vi "Add Bad Input Error.vi"(4 "missing value":string, 6 "name":string, 8 "error in":errorcluster, 10 "in connections map":bool) -> (0 "error out":errorcluster)   [LabVIEW 2020, in "MeasurementLink Session Management.lvlib" / "Session Reservation.lvclass"]
uses:
  Session Reservation.lvclass
  MeasurementLink Measurement Server/Helpers/Error Strings Global Internal.vi
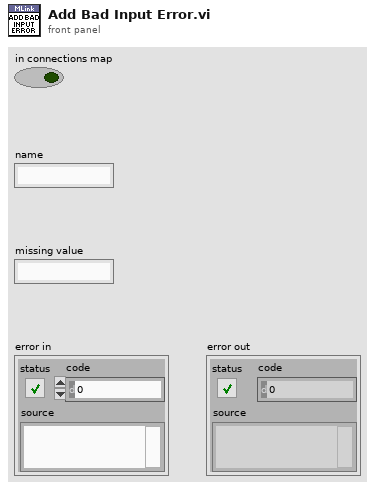
[diagram p1: front panel]
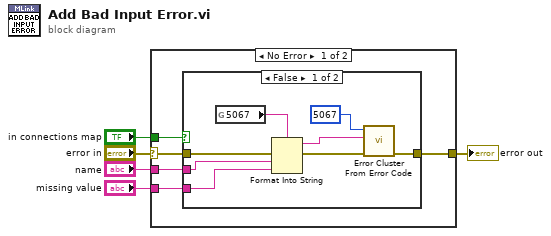
[diagram p0: block diagram]
diagram:
  n1 = case shown="No Error" "error in" {
    selector: "error in" -> [w8 w20]
    tunnel: "missing value" -> [w10 _]
    tunnel: "in connections map" -> [w9 _]
    tunnel: [w7 w20] -> w2
    tunnel: "name" -> [w6 _]
    frame No Error {
      n2 = case shown="False" w9 {
        tunnel: [w18 w19] -> w7
        tunnel: w8 -> [w16 w19]
        tunnel: w10 -> [w12 _]
        tunnel: w6 -> [w11 _]
        frame False {
          n3 = global read "Error Strings Global Internal.vi" "5067"() -> (w17:string)
          n4 = Format Into String(format string=w17, error in=w16, w11, w12) -> (resulting string=w13:string, error out=w15:errorcluster)  [unwired: 1 in]
          n5 = call <vilib>:"Error Cluster From Error Code.vi"("error in (no error)"=w15, "error message (\"\")"=w13, "error code (0)"=5067) -> ("error out"=w18:errorcluster)  [unwired: 6 in]
        }
        frame True {
        }
      }
    }
    frame Error {
    }
  }
  "error out" <- w2
